vi "CaratteristicaDinamica -simulato.vi"() -> ()   [LabVIEW 2018]
uses:
  <vilib>/Analysis/baseanly.llb/Mean (DBL).vi
  <vilib>/Analysis/5stat.llb/RMS (DBL).vi
  <vilib>/Waveform/WDTFileIO.llb/Read Waveform from File.vi
  <vilib>/measure/matone.llb/SINAD Analyzer 1 Chan.vi
  <vilib>/measure/NI_MAPro.lvlib
  <vilib>/Analysis/NI_AALPro.lvlib
  <vilib>/Analysis/NI_AALBase.lvlib
panel:
  out "SNR":dbl=49.64994620708113
  in  "Tab Control":T1(tab)=enum."ANDAMENTO ENOB"
  out "Confronto":waveform(dbl)[](graph)=[{"t0"=timestamp(0 s since 1904-01-01), "dt"=2.0000000233721948e-07, "Y"=array[14000 elements]}, {"t0"=timestamp(0 s since 1904-01-01), "dt"=2.0000000233721948e-07, "Y"=array[14000 elements]}]
  out "noise":waveform(dbl)(graph)={"t0"=timestamp(0 s since 1904-01-01), "dt"=2.0000000233721948e-07, "Y"=array[14000 elements]}
  out "rumore a media nulla":waveform(dbl)(graph)={"t0"=timestamp(0 s since 1904-01-01), "dt"=2.0000000233721948e-07, "Y"=array[14000 elements]}
  out "ENOB-FREQ":cluster{dbl[], dbl[]}(graph)={[100.0, 1000.0, 10000.0, 100000.0, 1000000.0, 10000000.0], [5.45766, 5.53013, 5.48815, 5.42602, 5.10374, 4.74128]}
  in  "file path (dialog if empty)":path=path "E:/Documenti/OneDrive - Universita' degli Studi della Campania Luigi Vanvitelli/Università/2 Magistrale/Laboratorio/progetto/GRUPPO C/CaratteristicaDinamicaADC/simulazioni/dinamica 1k"
  out "ENOB":dbl=6.760950212118806
  # "PARAMETRI DELL'ADC"
  # "FREQUENZA"
  # "ENOB"
  # "5,45766"
  # "100 Hz"
  # "5,53013"
  # "1kHz"
  # "10kHz"
  # "5,48815"
  # "100kHz"
  # "5,42602"
  # "1MHz"
  # "5,10374"
  # "10MHz"
  # "4,74128"
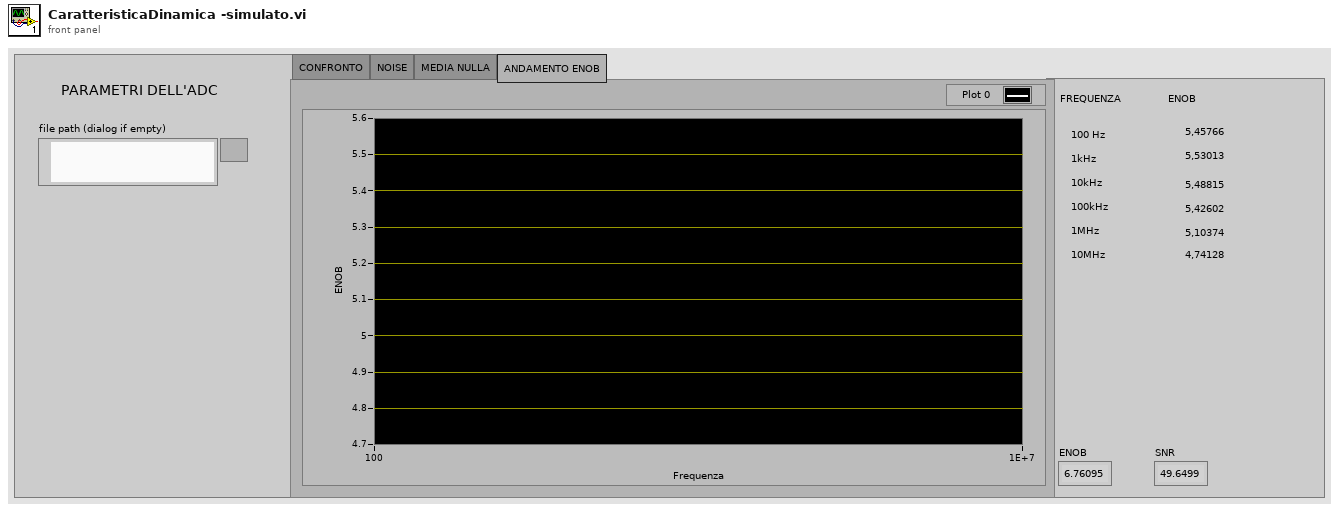
[diagram p1: front panel]
types:
  T1 = enum32{"CONFRONTO", "NOISE", "MEDIA NULLA", "ANDAMENTO ENOB"}
  T2 = enum16{"none", "input signal", "fundamental signal", "residual signal"}
  T3 = cluster{"exported time signal":waveform(dbl), "exported spectrum (dB)":cluster{"f0":dbl, "df":dbl, "dB Spectrum (Hann)":dbl[]}}
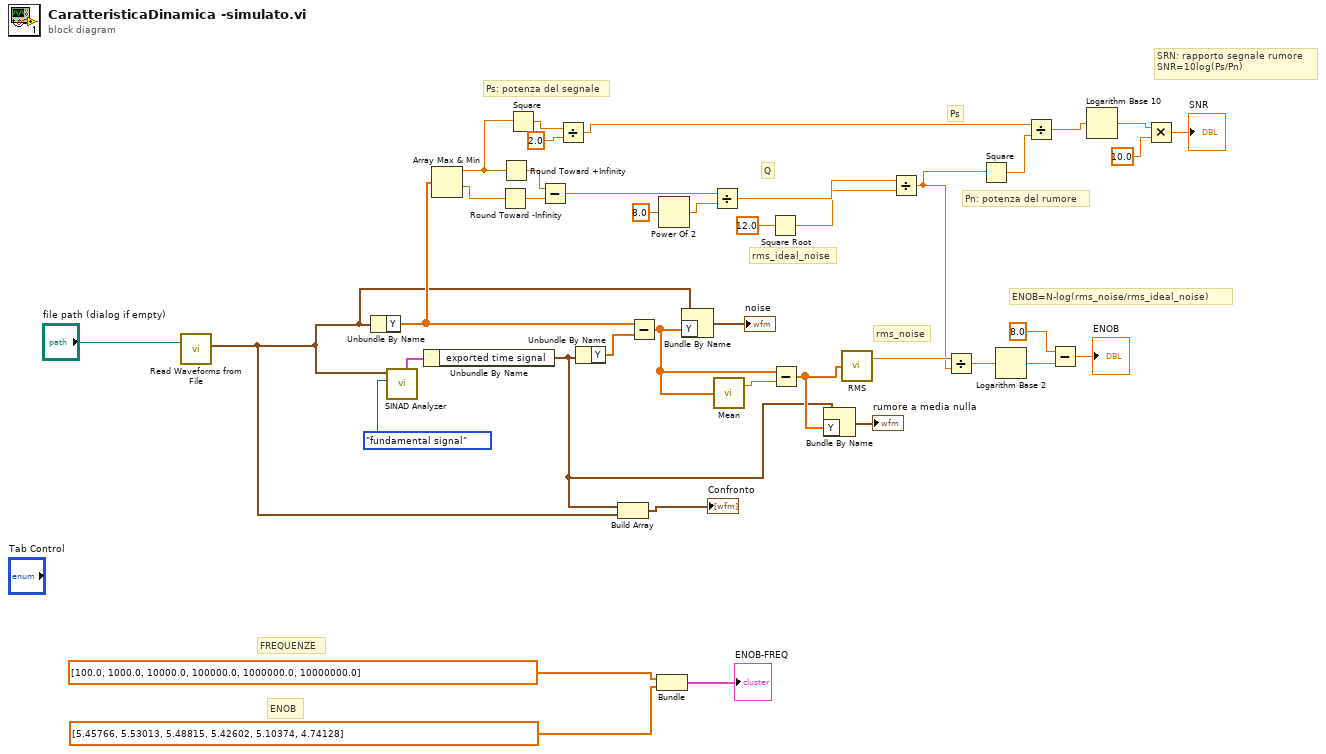
[diagram p0: block diagram]
diagram:
  # "SRN: rapporto segnale rumore\nSNR=10log(Ps/Pn)"
  # "Ps"
  # "Ps: potenza del segnale"
  # "Pn: potenza del rumore"
  # "FREQUENZE"
  # "ENOB"
  # "ENOB=N-log(rms_noise/rms_ideal_noise)"
  # "rms_noise"
  # "rms_ideal_noise"
  # "Q"
  n1 = call-poly <vilib>:"Read Waveforms from File.vi"("file path (dialog if empty)"="file path (dialog if empty)") -> ("first waveform in record"=w2:waveform(dbl))  [unwired: 5 in, 3 out]
  n2 = Unbundle By Name(w2) -> ("Y"=w36:dbl[])
  n3 = call-poly <vilib>:"SINAD Analyzer.vi"("export  mode"=T2."fundamental signal", "signal in"=w2) -> ("exported signals"=w39:T3)  [unwired: 4 in, 5 out]
  n4 = Unbundle By Name(w39) -> ("exported time signal"=w1:waveform(dbl))
  n5 = Array Max & Min(array=w36) -> (max value=w16:dbl, min value=w18:dbl)  [unwired: 2 out]
  n6 = Round Toward -Infinity(1:w18) -> (0:w17:dbl)
  n7 = Round Toward +Infinity(x=w16) -> (ceil(x): smallest int >= x=w19:dbl)
  n8 = Square(x=w16) -> (x^2=w15:dbl)
  n9 = Subtract(x=w19, y=w17) -> (x-y=w35:dbl)
  n10 = Divide(x=w15, y=2.0) -> (x/y=w12:dbl)
  n11 = Unbundle By Name(w1) -> ("Y"=w38:dbl[])
  n12 = Build Array(w1, w2) -> (→"Confronto":waveform(dbl)[])
  n13 = Subtract(x=w36, y=w38) -> (x-y=w5:dbl[])
  n14 = Bundle(dbl[] [100.0, 1000.0, 10000.0, 100000.0, 1000000.0, 10000000.0], dbl[] [5.45766, 5.53013, 5.48815, 5.42602, 5.10374, 4.74128]) -> (→"ENOB-FREQ":cluster{dbl[], dbl[]})  [unwired: 1 in]
  n15 = Power Of 2(x=8.0) -> (2^x=w34:dbl)
  n16 = Bundle By Name(cluster=w2, "Y"=w5) -> (→"noise":waveform(dbl))
  n17 = Divide(x=w35, y=w34) -> (x/y=w33:dbl)
  n18 = call-poly <vilib>:"Mean.vi"("X"=w5) -> ("mean"=w6:dbl)  [unwired: 1 out]
  n19 = Square Root(x=12.0) -> (sqrt(x)=w32:dbl)
  n20 = Subtract(x=w5, y=w6) -> (x-y=w4:dbl[])
  n21 = Bundle By Name(cluster=w1, "Y"=w4) -> (→"rumore a media nulla":waveform(dbl))
  n22 = call-poly <vilib>:"RMS.vi"("X"=w4) -> ("rms value"=w30:dbl)  [unwired: 1 out]
  n23 = Divide(x=w33, y=w32) -> (x/y=w13:dbl)
  n24 = Divide(x=w30, y=w13) -> (x/y=w29:dbl)
  n25 = Square(x=w13) -> (x^2=w11:dbl)
  n26 = Logarithm Base 2(1:w29) -> (0:w26:dbl)
  n27 = Divide(x=w12, y=w11) -> (x/y=w10:dbl)
  n28 = Subtract(x=8.0, y=w26) -> (x-y=→"ENOB":dbl)
  n29 = Logarithm Base 10(1:w10) -> (0:w9:dbl)
  n30 = Multiply(x=w9, y=10.0) -> (x*y=→"SNR":dbl)
